vi "niUSRP EX FSK Tx.vi"() -> ()   [LabVIEW 2018]
doc: "This example <B>requires the Modulation Toolkit</B>.\n\nApplies Frequency Shift Keying (FSK) to a PN sequence for USRP-based transmission. Continuously transmits a repeating message with a length determined by the PN Sequence Order parameter. \n\nThe example can generate FSK formats including 2-, 4-, 8-, and 16-FSK. It applies a pulse-shaping filter to the message signal, resamples the data to suit the timing specifications of the AWG, and ensures phase continuity in the data. \n\nYou can adjust the Digital Up Converter (DUC) Pre-Filter Gain to avoid overflow."
uses:
  <vilib>/addons/Modulation/Digital/General/MT Generate FSK System Parameters(M).vi
  <instrlib>/niUSRP/niUSRP Write Tx Data (CDB Cluster).vi
  <vilib>/addons/Modulation/niDMT.lvlib
panel:
  in  "Enabled Channel":string(combo)="0"
  out "Tx Gain [dB] (actual)":dbl format="%#.6p"
  out "Tx Frequency \n[Hz] (actual)":dbl format="%#.6p"
  out "Tx IQ Sampling\nRate [S/sec] (actual)":dbl format="%#.6p"
  in  "Active Antenna":string(combo)="TX1"
  in  "Tx Gain [dB]":dbl format="%#.6p"
  in  "Tx Frequency\n[Hz]":dbl=915000000.0 format="%#.6p"
  in  "Tx IQ Sampling\nRate [S/sec]":dbl=200000.0 format="%#.6p"
  in  "Device Name":refnum<k15>="192.168.10.2"
  in  "Filter Parameters":T1={"Alpha"=0.5, "Filter Length"=4, "TX Filter"=enum."Gaussian"} caption="Pulse Shaping Filter Parameters" {"Alpha" format="%.2f"}
  in  "Fsk M-Ary":T2(ring)
  out "Signal Bandwidth [Hz]":dbl=166666.6666666667 format="%#.2p"
  in  "Specify Mode":T3(tab)=enum."Specify FSK Deviation"
  in  "Modulation Index":dbl=0.3 format="%.2f"
  in  "FSK Deviation":dbl=50000.0 format="%#.4p"
  out "Generating?":bool
  in  "Stop":bool
  in  "Samples Per Symbol":i32=4
  out "Symbol Rate [Hz]":dbl=44444.444444444445 format="%#.2p"
  in  "Pn Sequence Order":i32=13 min=5 max=16 step=1
  out "error out":errorcluster
  out "Frequency Deviation [Hz]":dbl=50000.0 format="%#.4p"
  # "FSK  Parameters"
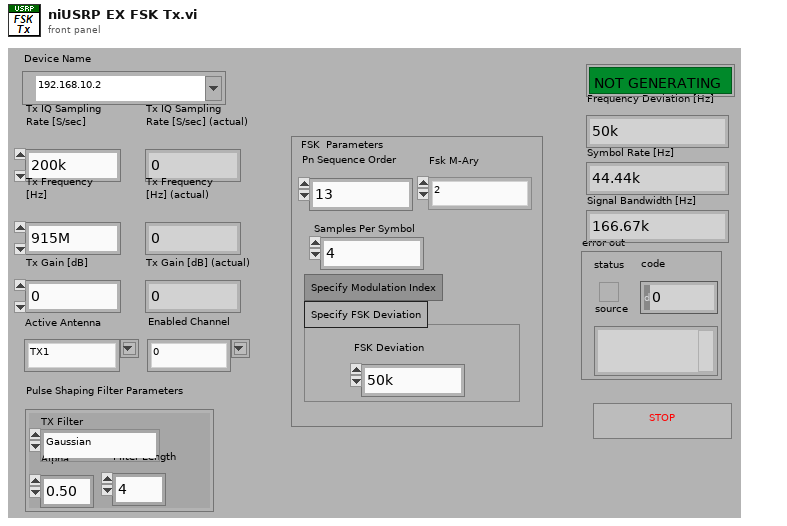
[diagram p1: front panel]
types:
  T1 = cluster{"Alpha":dbl, "Filter Length":i32, "TX Filter":enum16{"none", "Raised Cosine", "Root Raised Cos", "Gaussian"}}
  T2 = enum16{"2", "4", "8", "16", "32", "64", "128", "256"}
  T3 = enum32{"Specify Modulation Index", "Specify FSK Deviation"}
  T4 = enum16{"none", "Raised Cosine", "Root Raised Cos", "Gaussian"}
  T5 = cluster{"samples per symbol (16)":i32, "symbol map":dbl[], "symbol phase continuity":enum16{"continuous", "discontinuous"}}
  T6 = typedef "niAMT.lvlib/Complex Data Waveform.ctl" = cluster{"t0":dbl, "dt":dbl, "Y":cdb[]}
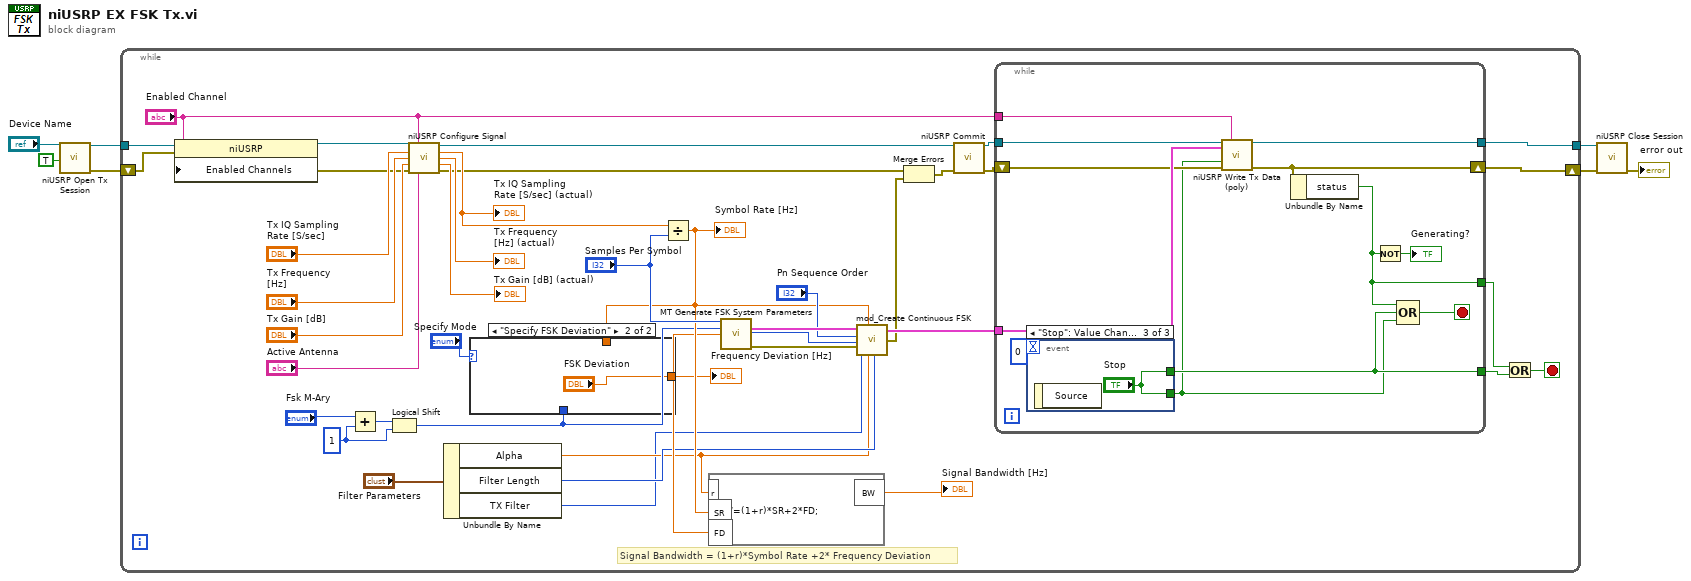
[diagram p0: block diagram]
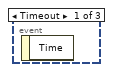
[diagram p2: hidden frame]
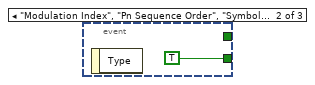
[diagram p3: hidden frame]
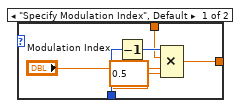
[diagram p4: hidden frame]
diagram:
  n1 = call <instrlib>:"niUSRP Open Tx Session.vi"("device names"="Device Name", "reset"=TRUE) -> ("session handle out"=w5:refnum<k15>, "error out"=w4:errorcluster)  [unwired: 12 in]
  n2 = while {
    tunnel: w5 -> [w15]
    tunnel: [w27] -> w2
    shift-right: [w40] -> w1
    shift-left: w4 -> [w14]
    stop <- w46 stop-if-true
    w36 = 1
    # "Signal Bandwidth = (1+r)*Symbol Rate +2* Frequency Deviation"
    n3 = property class="niUSRP"(reference=w15, error in=w14, "Enabled Channels"="Enabled Channel") -> (reference out=w13:refnum<k15>, error out=w12:errorcluster)
    n4 = Add(x="Fsk M-Ary", y=w36) -> (x+y=w37:i32)
    n5 = Logical Shift(y=w37, x=w36) -> (x << y=w20:i32)
    n6 = call <instrlib>:"niUSRP Configure Signal.vi"("session handle"=w13, "channel list"="Enabled Channel", "IQ rate"="Tx IQ Sampling\nRate [S/sec]", "carrier frequency"="Tx Frequency\n[Hz]", "gain"="Tx Gain [dB]", "error in (no error)"=w12, "active antenna"="Active Antenna") -> ("session handle out"=w18:refnum<k15>, "coerced IQ rate"=w19:dbl, "coerced carrier frequency"=→"Tx Frequency \n[Hz] (actual)":dbl, "coerced gain"=→"Tx Gain [dB] (actual)":dbl, "error out"=w9:errorcluster)  [unwired: 4 in]
    "Tx IQ Sampling\nRate [S/sec] (actual)" <- w19
    n7 = Unbundle By Name("Filter Parameters") -> ("Alpha"=w30:dbl, "Filter Length"=w31:i32, "TX Filter"=w29:T4)
    n8 = Divide(x=w19, y="Samples Per Symbol") -> (x/y=w34:dbl)
    "Symbol Rate [Hz]" <- w34
    n9 = case shown="\"Specify FSK Deviation\"" "Specify Mode" {
      tunnel: w34 -> [w67 _]
      tunnel: [w66 "FSK Deviation"] -> w33
      tunnel: w20 -> [w64 _]
      frame "Specify Modulation Index", Default {
        n10 = Decrement(x=w64) -> (x-1=w68:i32)
        n11 = Compound Arithmetic op=MULTIPLY(w68, w67, "Modulation Index", 0.5 ("value")) -> (w66:dbl)
      }
      frame "Specify FSK Deviation" {
      }
    }
    "Frequency Deviation [Hz]" <- w33
    n12 = formula code="BW=(1+r)*SR+2*FD;"("r"=w30, "SR"=w34, "FD"=w33) -> ("BW"=→"Signal Bandwidth [Hz]":dbl)
    n13 = call-poly <vilib>:"MT Generate FSK System Parameters.vi"("samples per symbol (16)"="Samples Per Symbol", "M-FSK (2)"=w20, "FSK deviation (Hz)"=w33) -> ("FSK system parameters"=w48:T5, "bits per symbol"=w45:i32, "error out"=w41:errorcluster)  [unwired: 10 in]
    n14 = call <vilib>:"mod_Create Continuous FSK.vi"("Filter Length"=w31, "TX Filter"=w29, "BT"=w30, "error in (no error)"=w41, "bits per symbol"=w45, "Symbol Rate, Hz"=w34, "PN Sequence Order"="Pn Sequence Order", "FSK system parameters"=w48) -> ("error out"=w10:errorcluster, "output complex waveform"=w42:T6)  [unwired: 1 out]
    n15 = Merge Errors(w9, w10) -> (w8:errorcluster)
    n16 = call <instrlib>:"niUSRP Commit.vi"("session handle"=w18, "error in (no error)"=w8) -> ("session handle out"=w17:refnum<k15>, "error out"=w16:errorcluster)  [unwired: 12 in]
    n17 = while {
      shift-right: [w49] -> w40
      shift-left: w16 -> [w54]
      tunnel: [w55] -> w39
      tunnel: [w50] -> w47
      tunnel: w42 -> [w57]
      tunnel: w17 -> [w58]
      tunnel: [w56] -> w27
      tunnel: "Enabled Channel" -> [w52]
      stop <- w60 stop-if-true
      n18 = event shown="[2] \"Stop\": Value Change" {
        selector: _ -> [_ _ _]
        dyn-events: _ -> [_ _ _]
        timeout: 0 -> [_ _ _]
        tunnel: [_ TRUE "Stop"] -> w53
        tunnel: [_ _ "Stop"] -> w55
        event Timeout {
          n19 = event-data() -> ()  [unwired: 1 in, 1 out]
        }
        event "Modulation Index", "Pn Sequence Order", "Symbol Rate [Hz]", "Samples Per Symbol", "Specify Mode", "Fsk M-Ary", "Filter Parameters", "Tx Frequency\n[Hz]", "Tx IQ Sampling\nRate [S/sec]", "Tx Gain [dB]", "Active Antenna", "FSK Deviation": Value Change {
          n20 = event-data() -> ()  [unwired: 1 in, 1 out]
        }
        event "Stop": Value Change {
          n21 = event-data() -> ()  [unwired: 1 in, 1 out]
        }
      }
      n22 = call-poly <instrlib>:"niUSRP Write Tx Data (poly).vi"("session handle"=w58, "channel list"=w52, "data"=w57, "end of data?"=w53, "error in (no error)"=w54) -> ("session handle out"=w56:refnum<k15>, "error out"=w49:errorcluster)  [unwired: 9 in]
      n23 = Unbundle By Name(w49) -> ("status"=w50:bool)
      n24 = Not(x=w50) -> (.not. x?=→"Generating?":bool)
      n25 = Compound Arithmetic op=OR(w50, w55, w53) -> (w60:bool)
    }
    n26 = Or(x=w47, y=w39) -> (x .or. y?=w46:bool)
  }
  n27 = call <instrlib>:"niUSRP Close Session.vi"("session handle"=w2, "error in (no error)"=w1) -> ("error out"=→"error out":errorcluster)  [unwired: 13 in]
